vi "MCP3422 Read 3 bytes.vi"(0 "VISA Refnum in":refnum<visa-resource-name>, 11 "error in (no error)":errorcluster) -> (4 "VISA Refnum out":refnum<visa-resource-name>, 6 "1st data byte":u8, 8 "2nd data byte":u8, 10 "configuration byte":u8, 15 "error out":errorcluster)   [LabVIEW 2015]
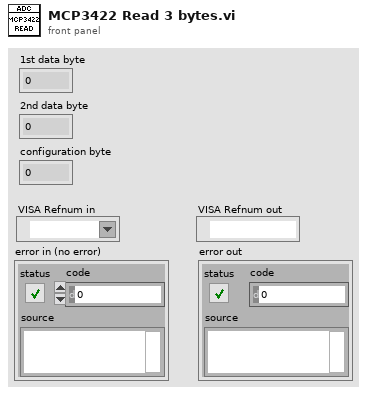
[diagram p1: front panel]
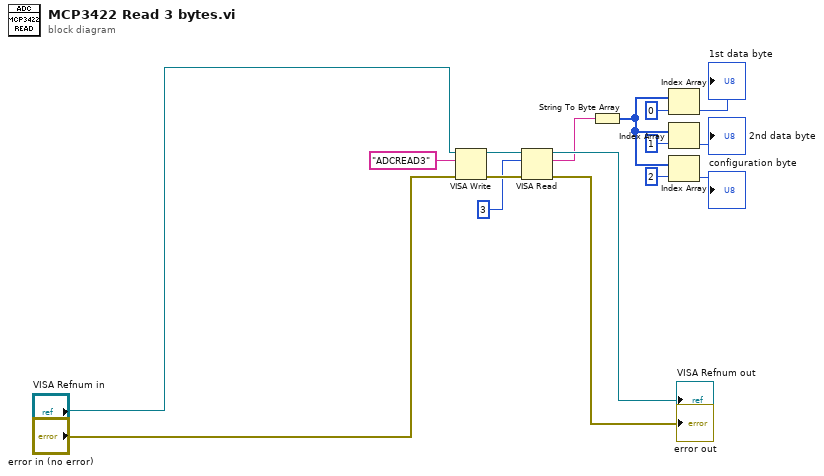
[diagram p0: block diagram]
diagram:
  n1 = VISA Write(VISA resource name="VISA Refnum in", write buffer="ADCREAD3", error in (no error)="error in (no error)") -> (VISA resource name out=w14:refnum<visa-resource-name>, error out=w13:errorcluster)  [unwired: 1 out]
  n2 = VISA Read(VISA resource name=w14, byte count=u32 3, error in (no error)=w13) -> (VISA resource name out=→"VISA Refnum out":refnum<visa-resource-name>, read buffer=w9:string, error out=→"error out":errorcluster)  [unwired: 1 out]
  n3 = String To Byte Array(string=w9) -> (unsigned byte array=w5:u8[])
  n4 = Index Array(array=w5, index=0) -> (element=→"1st data byte":u8)
  n5 = Index Array(array=w5, index=1) -> (element=→"2nd data byte":u8)
  n6 = Index Array(array=w5, index=2) -> (element=→"configuration byte":u8)
